vi "line and page break constant.vi"() -> (0 "line and page breaks":T1={"Widow/orphan ctrl"=2, "Keeps lines together"=0, "Keep with next"=0, "Page break before"=0, "Suppress line numbers"=0, "Don't hyphenate"=0} {"Don't hyphenate" items=["Unchanged", "No", "Yes"]; "Suppress line numbers" items=["Unchanged", "No", "Yes"]; "Page break before" items=["Unchanged", "No", "Yes"]; "Keep with next" items=["Unchanged", "No", "Yes"]; "Keeps lines together" items=["Unchanged", "No", "Yes"]; "Widow/orphan ctrl" items=["Unchanged", "No", "Yes"]})   [LabVIEW 2010, in "NI_ReportGenerationToolkit.lvlib"]
doc: "Defines line and page break attributes of a specified range within a document."
uses:
  <vilib>/addons/_office/NI_ReportGenerationToolkit.lvlib
panel:
  # "Pagination"
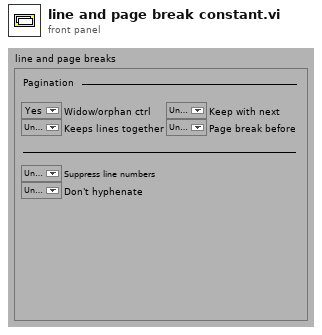
[diagram p1: front panel]
types:
  T1 = cluster{"Widow/orphan ctrl":u16, "Keeps lines together":u16, "Keep with next":u16, "Page break before":u16, "Suppress line numbers":u16, "Don't hyphenate":u16}
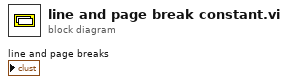
[diagram p0: block diagram]
diagram:
